vi "Load Players From File.vi"(11 "Path":path) -> (3 "Array":string[](array[string]))   [LabVIEW 2014]
uses:
  <vilib>/Utility/file.llb/Read From Spreadsheet File (string).vi
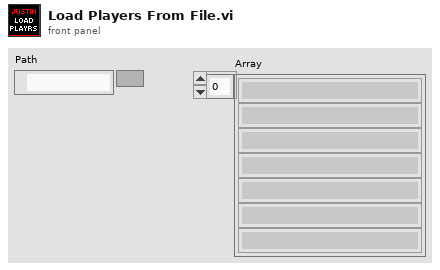
[diagram p1: front panel]
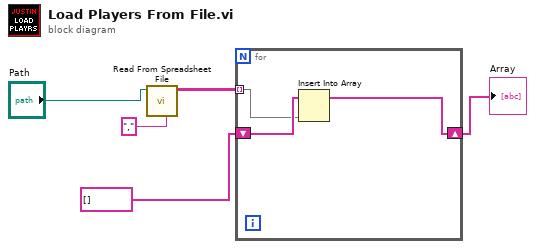
[diagram p0: block diagram]
diagram:
  n1 = call-poly <vilib>:"Read From Spreadsheet File.vi"("delimiter (\\t)"="," ("delimiter (\\t)"), "file path (dialog if empty)"="Path") -> ("all rows"=w3:string[][])  [unwired: 5 in, 4 out]
  n2 = for {
    tunnel: w3 -> [w7] mode=indexing
    shift-right: [w6] -> w1
    shift-left: string[] [] -> [w8]
    n3 = Insert Into Array(array=w8, new element=w7) -> (w6:string[])  [unwired: 1 in]
  }
  "Array" <- w1
